vi "Measurement.Uninit.vi"(8 "error in (no error)":errorcluster, 11 "Measurement.Free in":refnum<class "Measurement.Free.lvclass">) -> (0 "error out":errorcluster, 3 "Measurement.Free out":refnum<class "Measurement.Free.lvclass">)   [LabVIEW 2019, in "Measurement.Free.lvclass"]
uses:
  Measurement.Free.lvclass
  MC/MC.lvclass
  E:/UPWORK/Laser Tool/Laser/project/Subsystems/Device/Device.lvclass
  OPA/OPA.lvclass
  OPM/OPM.lvclass
  LIA/LIA.lvclass
  SMU/SMU.lvclass
  Device/Device.lvclass
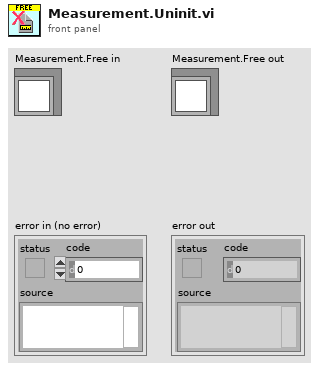
[diagram p1: front panel]
types:
  T1 = typedef "Measurement.Free.lvclass/Configuration--Cluster.ctl" = cluster{"Measurement.Type":T2, "Hardware":T3}
  T2 = typedef "Measurement.lvclass/Measurement.Type--Enum.ctl" = enum16{"Free", "I/V Curve", "Wavelength sweeping", "Photocurrent mapping"}
  T3 = typedef "Measurement.Free.lvclass/Configuration.Hardware--Cluster.ctl" = cluster{"SMU":T4, "LIA":T6, "OPM":T8, "OPA":T10, "MC":T12}
  T4 = typedef "Measurement.lvclass/Configuration.SMU--Cluster.ctl" = cluster{"Enable":bool, "SMU Model":string, "Configuration":T5}
  T5 = typedef "SMU.lvclass/Configuration--Cluster.ctl" = cluster{"VISA Resource":string, "Channel":string}
  T6 = typedef "Measurement.lvclass/Configuration.LIA--Cluster.ctl" = cluster{"Enable":bool, "LIA Model":string, "Configuration":T7}
  T7 = typedef "LIA.lvclass/Configuration--Cluster.ctl" = cluster{"VISA Resource":string}
  T8 = typedef "Measurement.lvclass/Configuration.OPM--Cluster.ctl" = cluster{"Enable":bool, "OPM Model":string, "Configuration":T9}
  T9 = typedef "OPM.lvclass/Configuration--Cluster.ctl" = cluster{"VISA Resource":string}
  T10 = typedef "Measurement.lvclass/Configuration.OPA--Cluster.ctl" = cluster{"Enable":bool, "OPA Model":string, "Configuration":T11}
  T11 = typedef "OPA.lvclass/Configuration--Cluster.ctl" = cluster{"Serial Number":string}
  T12 = typedef "Measurement.lvclass/Configuration.MC--Cluster.ctl" = cluster{"Enable":bool, "MC Model":string, "Configuration":T13}
  T13 = typedef "MC.lvclass/Configuration--Cluster.ctl" = cluster{"VISA Resource":string}
  T14 = typedef "Measurement.Free.lvclass/Dependencies--Cluster.ctl" = cluster{"SMU":refnum<class "SMU.lvclass">, "LIA":refnum<class "LIA.lvclass">, "OPM":refnum<class "OPM.lvclass">, "OPA":refnum<class "OPA.lvclass">, "MC":refnum<class "MC.lvclass">}
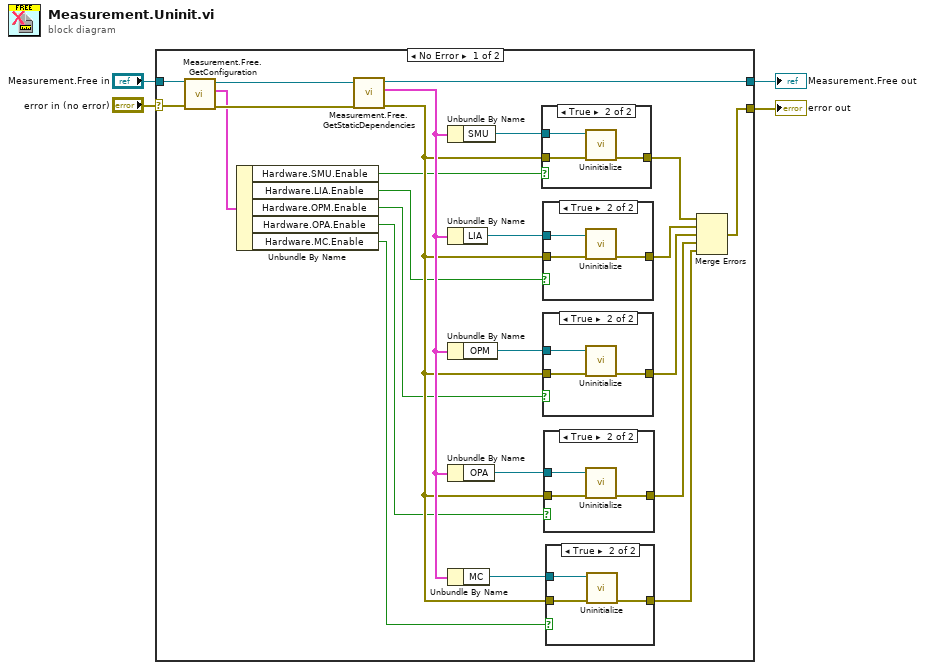
[diagram p0: block diagram]
diagram:
  n1 = case shown="No Error" "error in (no error)" {
    selector: "error in (no error)" -> [w12 w50]
    tunnel: [w25 w50] -> w1
    tunnel: [w27 w49] -> w2
    tunnel: "Measurement.Free in" -> [w14 w49]
    frame No Error {
      n2 = call "Measurement.Free.GetConfiguration.vi"("error in (no error)"=w12, "Measurement.Free"=w14) -> ("error out"=w11:errorcluster, "Configuration"=w10:T1, "Measurement.Free out"=w13:refnum<class "Measurement.Free.lvclass">)  [unwired: 7 in]
      n3 = Unbundle By Name(w10) -> ("Hardware.SMU.Enable"=w9:bool, "Hardware.LIA.Enable"=w8:bool, "Hardware.OPM.Enable"=w7:bool, "Hardware.OPA.Enable"=w6:bool, "Hardware.MC.Enable"=w5:bool)
      n4 = call "Measurement.Free.GetStaticDependencies.vi"("error in (no error)"=w11, "Measurement.Free"=w13) -> ("error out"=w15:errorcluster, "Dependencies"=w18:T14, "Measurement.Free out"=w27:refnum<class "Measurement.Free.lvclass">)  [unwired: 7 in]
      n5 = Unbundle By Name(w18) -> ("SMU"=w28:refnum<class "SMU.lvclass">)
      n6 = Unbundle By Name(w18) -> ("LIA"=w24:refnum<class "LIA.lvclass">)
      n7 = Unbundle By Name(w18) -> ("OPM"=w22:refnum<class "OPM.lvclass">)
      n8 = Unbundle By Name(w18) -> ("OPA"=w20:refnum<class "OPA.lvclass">)
      n9 = Unbundle By Name(w18) -> ("MC"=w17:refnum<class "MC.lvclass">)
      n10 = case shown="True" w9 {
        tunnel: w28 -> [_ w48]
        tunnel: [w45 w47] -> w26
        tunnel: w15 -> [w45 w46]
        frame False {
        }
        frame True {
          n11 = call "Uninitialize.vi"("error in (no error)"=w46, "Device in"=w48) -> ("error out"=w47:errorcluster)  [unwired: 8 in, 1 out]
        }
      }
      n12 = case shown="True" w8 {
        tunnel: w24 -> [_ w44]
        tunnel: [w41 w43] -> w23
        tunnel: w15 -> [w41 w42]
        frame False {
        }
        frame True {
          n13 = call "Uninitialize.vi"("error in (no error)"=w42, "Device in"=w44) -> ("error out"=w43:errorcluster)  [unwired: 8 in, 1 out]
        }
      }
      n14 = case shown="True" w7 {
        tunnel: w22 -> [_ w40]
        tunnel: [w37 w39] -> w21
        tunnel: w15 -> [w37 w38]
        frame False {
        }
        frame True {
          n15 = call "Uninitialize.vi"("error in (no error)"=w38, "Device in"=w40) -> ("error out"=w39:errorcluster)  [unwired: 8 in, 1 out]
        }
      }
      n16 = case shown="True" w6 {
        tunnel: w20 -> [_ w36]
        tunnel: [w33 w35] -> w19
        tunnel: w15 -> [w33 w34]
        frame False {
        }
        frame True {
          n17 = call "Uninitialize.vi"("error in (no error)"=w34, "Device in"=w36) -> ("error out"=w35:errorcluster)  [unwired: 8 in, 1 out]
        }
      }
      n18 = case shown="True" w5 {
        tunnel: w17 -> [_ w32]
        tunnel: [w29 w31] -> w16
        tunnel: w15 -> [w29 w30]
        frame False {
        }
        frame True {
          n19 = call "Uninitialize.vi"("error in (no error)"=w30, "Device in"=w32) -> ("error out"=w31:errorcluster)  [unwired: 8 in, 1 out]
        }
      }
      n20 = Merge Errors(w26, w23, w21, w19, w16) -> (w25:errorcluster)
    }
    frame Error {
    }
  }
  "error out" <- w1
  "Measurement.Free out" <- w2
